vi "Pack Run Headless Msg.vi"(10 "Mediator Type":refnum<class "IMediator.lvclass">) -> (3 "Run Headless Msg":refnum<class "Run Headless Msg.lvclass">)   [LabVIEW 2017, in "RootModel.lvlib" / "Run Headless Msg.lvclass"]
doc: "This VI sends the message to an actor."
uses:
  Run Headless Msg.lvclass
  IMediator/IMediator/IMediator.lvclass
  Run Headless Msg.lvclass/Run Headless Msg.ctl
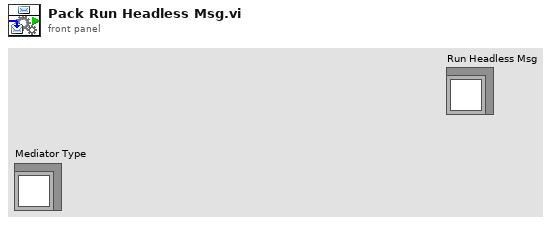
[diagram p1: front panel]
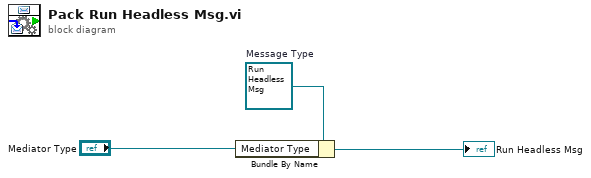
[diagram p0: block diagram]
diagram:
  w3 = refnum<class "Run Headless Msg.lvclass"> refnum  # Message Type
  n1 = Bundle By Name(cluster=w3, "Mediator Type"="Mediator Type") -> (→"Run Headless Msg":refnum<class "Run Headless Msg.lvclass">)
